vi "SVPO Peak Level (1 Ch DBL Array) with IC.vi"(6 "restart averaging? (F)":bool, 8 "initial conditions":T1={"historical max"=-inf, "historical min"=inf, "cumulative size"=0, "timestamp"=timestamp(0 s since 1904-01-01)}, 10 "sampling rate [Hz]":dbl=1.0, 11 "scaled signal [EU]":dbl[](array[numeric])) -> (0 "final conditions":T1, 1 "minimum level [EU]":dbl=nan, 2 "maximum level [EU]":dbl=nan, 3 "peak level [EU]":dbl=nan, 4 "duration [s]":dbl)   [LabVIEW 2017, in "SoundVib_VibrationLevel.lvlib"]
doc: "Uses a peak detector and computes the level of scaled time waveform signals and scaled array signals. <B>scaled signal [EU]</B> should have a zero DC component. You can attenuate the DC component with hardware AC-coupling filters and with software high-pass filters. Use this VI on embedded targets that have limited computational resources. Wire data to the scaled signal [EU] input to determine the polymorphic instance to use or manually select the instance."
uses:
  <vilib>/addons/Sound and Vibration/svt_Level/SoundVib_VibrationLevel.lvlib
  <vilib>/addons/_NISVFA/_Shared subVIs/Controls/svc_Peak Level State.ctl
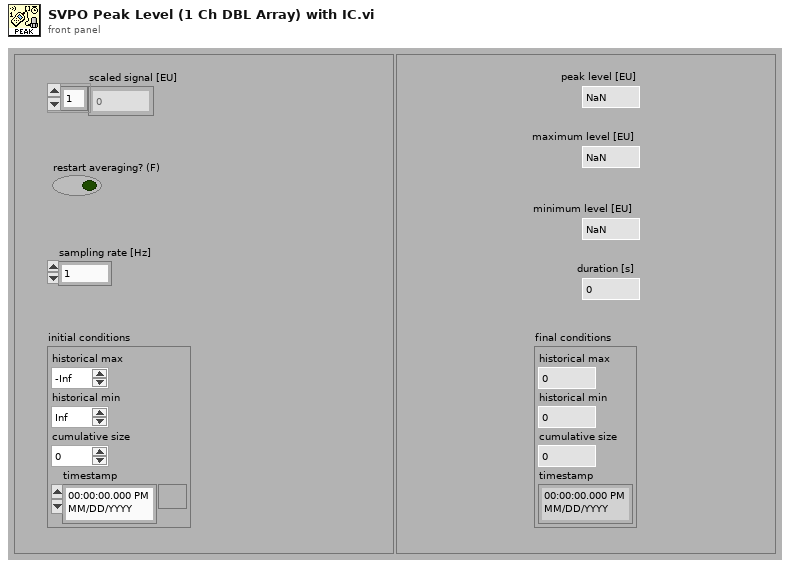
[diagram p1: front panel]
types:
  T1 = typedef "svc_Peak Level State.ctl" = cluster{"historical max":dbl, "historical min":dbl, "cumulative size":u64, "timestamp":timestamp}
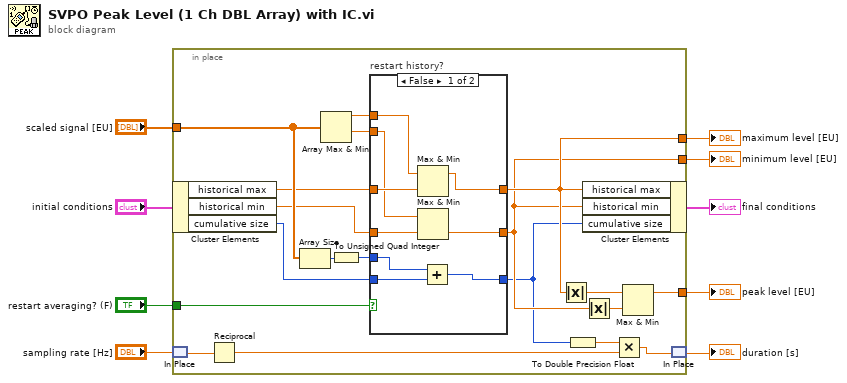
[diagram p0: block diagram]
diagram:
  n1 = in-place {
    in-place-border: "scaled signal [EU]" -> [w19]
    in-place-border: "restart averaging? (F)" -> [w10]
    in-place-border: [w15] -> w3
    in-place-border: [w14] -> w2
    in-place-border: [w13] -> w1
    n2 = in-place-cluster #1("initial conditions") -> ("historical max"=w18:dbl, "historical min"=w17:dbl, "cumulative size"=w16:u64)
    n3 = in-place-match #2("sampling rate [Hz]") -> (w27:dbl)
    n4 = Reciprocal(x=w27) -> (1/x=w28:dbl)
    n5 = Array Size(array=w19) -> (size(s)=w21:i32)
    n6 = Array Max & Min(array=w19) -> (max value=w24:dbl, min value=w25:dbl)  [unwired: 2 out]
    n7 = To Unsigned Quad Integer(1:w21) -> (0:w20:u64)
    n8 = case "restart history?" shown="False" w10 {
      tunnel: [w37 w38] -> w11
      tunnel: [w29 w39] -> w13
      tunnel: [w32 w40] -> w14
      tunnel: w18 -> [w33 _]
      tunnel: w17 -> [w30 _]
      tunnel: w16 -> [w36 _]
      tunnel: w25 -> [w31 w39]
      tunnel: w24 -> [w34 w40]
      tunnel: w20 -> [w35 w38]
      frame False {
        n9 = Max & Min(x=w34, y=w33) -> (max(x,y)=w32:dbl)  [unwired: 1 out]
        n10 = Max & Min(x=w31, y=w30) -> (min(x,y)=w29:dbl)  [unwired: 1 out]
        n11 = Add(x=w35, y=w36) -> (x+y=w37:u64)
      }
      frame True {
        # "no history: output\n current measurements"
      }
    }
    n12 = Absolute Value(x=w14) -> (abs(x)=w23:dbl)
    n13 = To Double Precision Float(number=w11) -> (double precision float=w12:dbl)
    n14 = in-place-cluster #1("historical max"=w14, "historical min"=w13, "cumulative size"=w11) -> (→"final conditions":T1)
    n15 = Absolute Value(x=w13) -> (abs(x)=w22:dbl)
    n16 = Multiply(x=w12, y=w28) -> (x*y=w26:dbl)
    n17 = Max & Min(x=w23, y=w22) -> (max(x,y)=w15:dbl)  [unwired: 1 out]
    n18 = in-place-match #2(w26) -> (→"duration [s]":dbl)
  }
  "peak level [EU]" <- w3
  "minimum level [EU]" <- w1
  "maximum level [EU]" <- w2
